vi "Sans titre 1.vi"() -> ()   [LabVIEW 2020]
uses:
  <vilib>/regexp/Match Regular Expression.xnode
panel:
  out "offset après correspondance":i32
  out "après la correspondance":string
  out "toute l'expression":string
  out "avant la correspondance":string
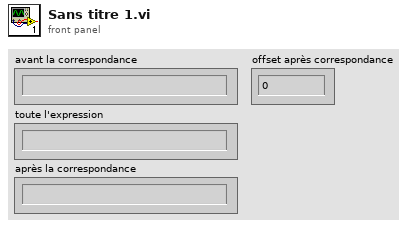
[diagram p1: front panel]
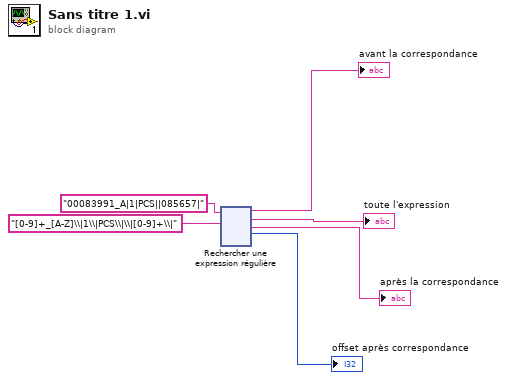
[diagram p0: block diagram]
diagram:
  n1 = xnode "Rechercher une expression régulière"("chaîne en entrée"="00083991_A|1|PCS||085657|", "expression régulière"="[0-9]+_[A-Z]\\|1\\|PCS\\|\\|[0-9]+\\|") -> ("avant la correspondance"=→"avant la correspondance":string, "toute l'expression"=→"toute l'expression":string, "après la correspondance"=→"après la correspondance":string, "offset après correspondance"=→"offset après correspondance":i32)  [unwired: 4 in, 1 out]
